vi "Send to Shell.vi"(7 "Session In":refnum<class "JuPyter_Client.lvclass">, 8 "error in (no error)":errorcluster, 10 "Parent Message":refnum<class "Message Class.lvclass">, 11 "object in":refnum<class "Request Message.lvclass">) -> (0 "error out":errorcluster, 2 "Reply Back":refnum<class "Reply Message.lvclass">, 3 "object out":refnum<class "Request Message.lvclass">, 5 "Session Out":refnum<class "JuPyter_Client.lvclass">)   [LabVIEW 2018, in "ClientMessaging.lvlib" / "Request Message.lvclass"]
doc: "Send this message to the shell socket on a session"
uses:
  Request Message.lvclass
  JuPyter_Client/JuPyter_Client.lvclass
  Message Class/Message Class.lvclass
  Reply Message/Reply Message.lvclass
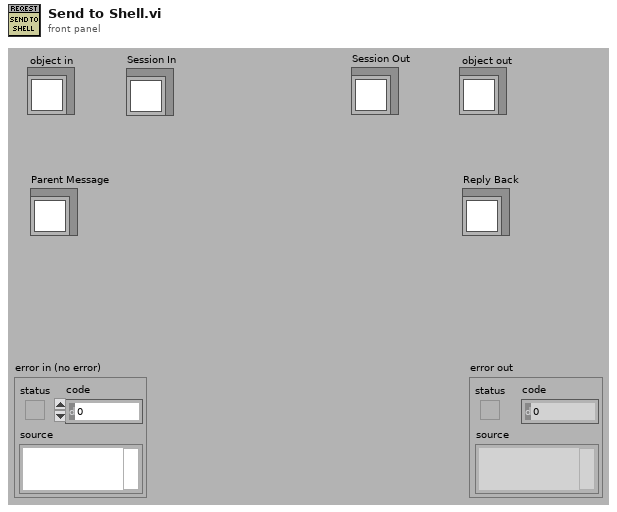
[diagram p1: front panel]
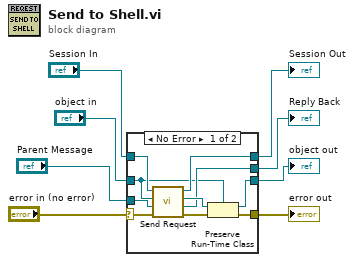
[diagram p0: block diagram]
diagram:
  n1 = case shown="No Error" "error in (no error)" {
    selector: "error in (no error)" -> [w13 w21]
    tunnel: [w9 w21] -> w7
    tunnel: [w12 w20] -> w5
    tunnel: "object in" -> [w11 w20]
    tunnel: "Session In" -> [w18 w19]
    tunnel: [w17 w19] -> w3
    tunnel: "Parent Message" -> [w15 _]
    tunnel: [w14 _] -> w1
    frame No Error {
      n2 = call-dynamic "Send Request.vi"("error in (no error)"=w13, "Parent Message"=w15, "Message to send"=w11, "object in"=w18) -> ("error out"=w10:errorcluster, "Reply Back"=w14:refnum<class "Reply Message.lvclass">, "Message Out"=w16:refnum<class "Request Message.lvclass">, "object out"=w17:refnum<class "JuPyter_Client.lvclass">)  [unwired: 4 in]
      n3 = Preserve Run-Time Class(object in=w16, error in=w10, 2:w11) -> (object out=w12:refnum<class "Request Message.lvclass">, error out=w9:errorcluster)
    }
    frame Error {
    }
  }
  "error out" <- w7
  "object out" <- w5
  "Session Out" <- w3
  "Reply Back" <- w1
